vi "Final GUI for Team RDA.vi"() -> ()   [LabVIEW 2022 SP3]
doc: "This example is used to make the attitude control"
uses:
  GUI Animation/Fan.ctl
  GUI Animation/Dial.ctl
  GUI Animation/WiFi.ctl
  <vilib>/Platform/TimedLoop/XDataNode/timing_clust.ctl
  <vilib>/Platform/TimedLoop/XDataNode/nitl_modes.ctl
  <vilib>/Platform/TimedLoop/XDataNode/wakeup.ctl
  <vilib>/platform/TimedLoop/XDataNode/XDataNode.xnode
  Attitude Indicator/lv-attitudecontrol.lvlib
  <vilib>/Platform/TimedLoop/XDataNode/XDNodeRunTimeDep.lvlib
panel:
  in  "Command Roll 2":dbl
  in  "Command Pitch 2":dbl
  out "Command Yaw2":dbl
  in  "MotorROn":bool
  in  "MotorLON":bool
  out "?":bool
  out "JoyButton":bool
  out "MotorRightThrottle":dbl
  out "MotorLeftThrottle":dbl
  in  "Command Roll":dbl
  in  "Command Pitch":dbl
  in  "Command Yaw":dbl
  in  "RightPWM":dbl
  in  "LeftPWM":dbl
  in  "Control2ESP":bool
  in  "State Machine":i8
  out "Dialog":string
  in  "PC2ESP":bool
  out "WiFi 2":T1
  out "WiFi":T1
  out "Throttle":T2 scale=0.0..100.0
  out "Right Propeller":T3
  out "Left Propeller":T3
  out "Boolean 6":bool
  out "Yaw Displayed":i16
  out "Roll Displayed":dbl
  out "Boolean 3":bool
  in  "stop 4":bool
  out "Boolean 2":bool
  in  "stop 3":bool
  out "Pitch Displayed":dbl
  in  "Yaw":dbl min=0.0 max=360.0
  in  "Roll":dbl min=-180.0 max=180.0
  in  "Pitch":dbl min=-90.0 max=90.0
  in  "Attitude Indicator":refnum<vi>(3d-picture)
  in  "stop":bool
  # "pitch and roll from control"
types:
  T1 = typedef "WiFi.ctl" = u16
  T2 = typedef "Dial.ctl" = dbl
  T3 = typedef "Fan.ctl" = bool
  T4 = typedef "lv-attitudecontrol.lvlib/AttitudeHandle.ctl" = cluster{"First Scene Object":refnum<vi>, "Drum":refnum<vi>, "Window":refnum<vi>, "Dial":refnum<vi>, "Scene Graph":refnum<vi>, "Last Drum Pitch":dbl, "Last Drum Roll ":dbl, "Last Dial Roll":dbl}
  T5 = typedef "XDNodeRunTimeDep.lvlib/timing_clust.ctl" = cluster{"Expected End [f-1]":u64, "Actual End [f-1]":u64, "Finished Late? [f-1]":bool, "Expected End [i-1]":u64, "Actual End [i-1]":u64, "Finished Late? [i-1]":bool, "Expected Start [i]":u64, "Actual Start [i]":u64, "Expected Start [f]":u64, "Actual Start [f]":u64, "Source Name":string, "Structure Name":string, "Period":i64, "Deadline":i64, "Offset":i64, "Start":i64, "Priority":i32, "Timeout":i32, "Mode":T6, "Wakeup Reason":T7, "Error":errorcluster, "Source Type":string, "Secondary Source Type":string, "Global End Time":u64, "Global Start Time":u64, "Frame Duration":u64, "Iteration Duration":u64, "Assigned CPU":i32, "I/O Scan Engine Mode":u32}
  T6 = typedef "XDNodeRunTimeDep.lvlib/nitl_modes.ctl" = enum32{"No Change", "Process missed periods, maintain original phase", "Discard missed periods, maintain original phase", "Process missed periods, ignore original phase", "Discard missed periods, ignore original phase"}
  T7 = typedef "XDNodeRunTimeDep.lvlib/wakeup.ctl" = enum32{"Normal", "Aborted", "Asynchronous wakeup", "Timing source error", "Timed loop error", "Timeout"}
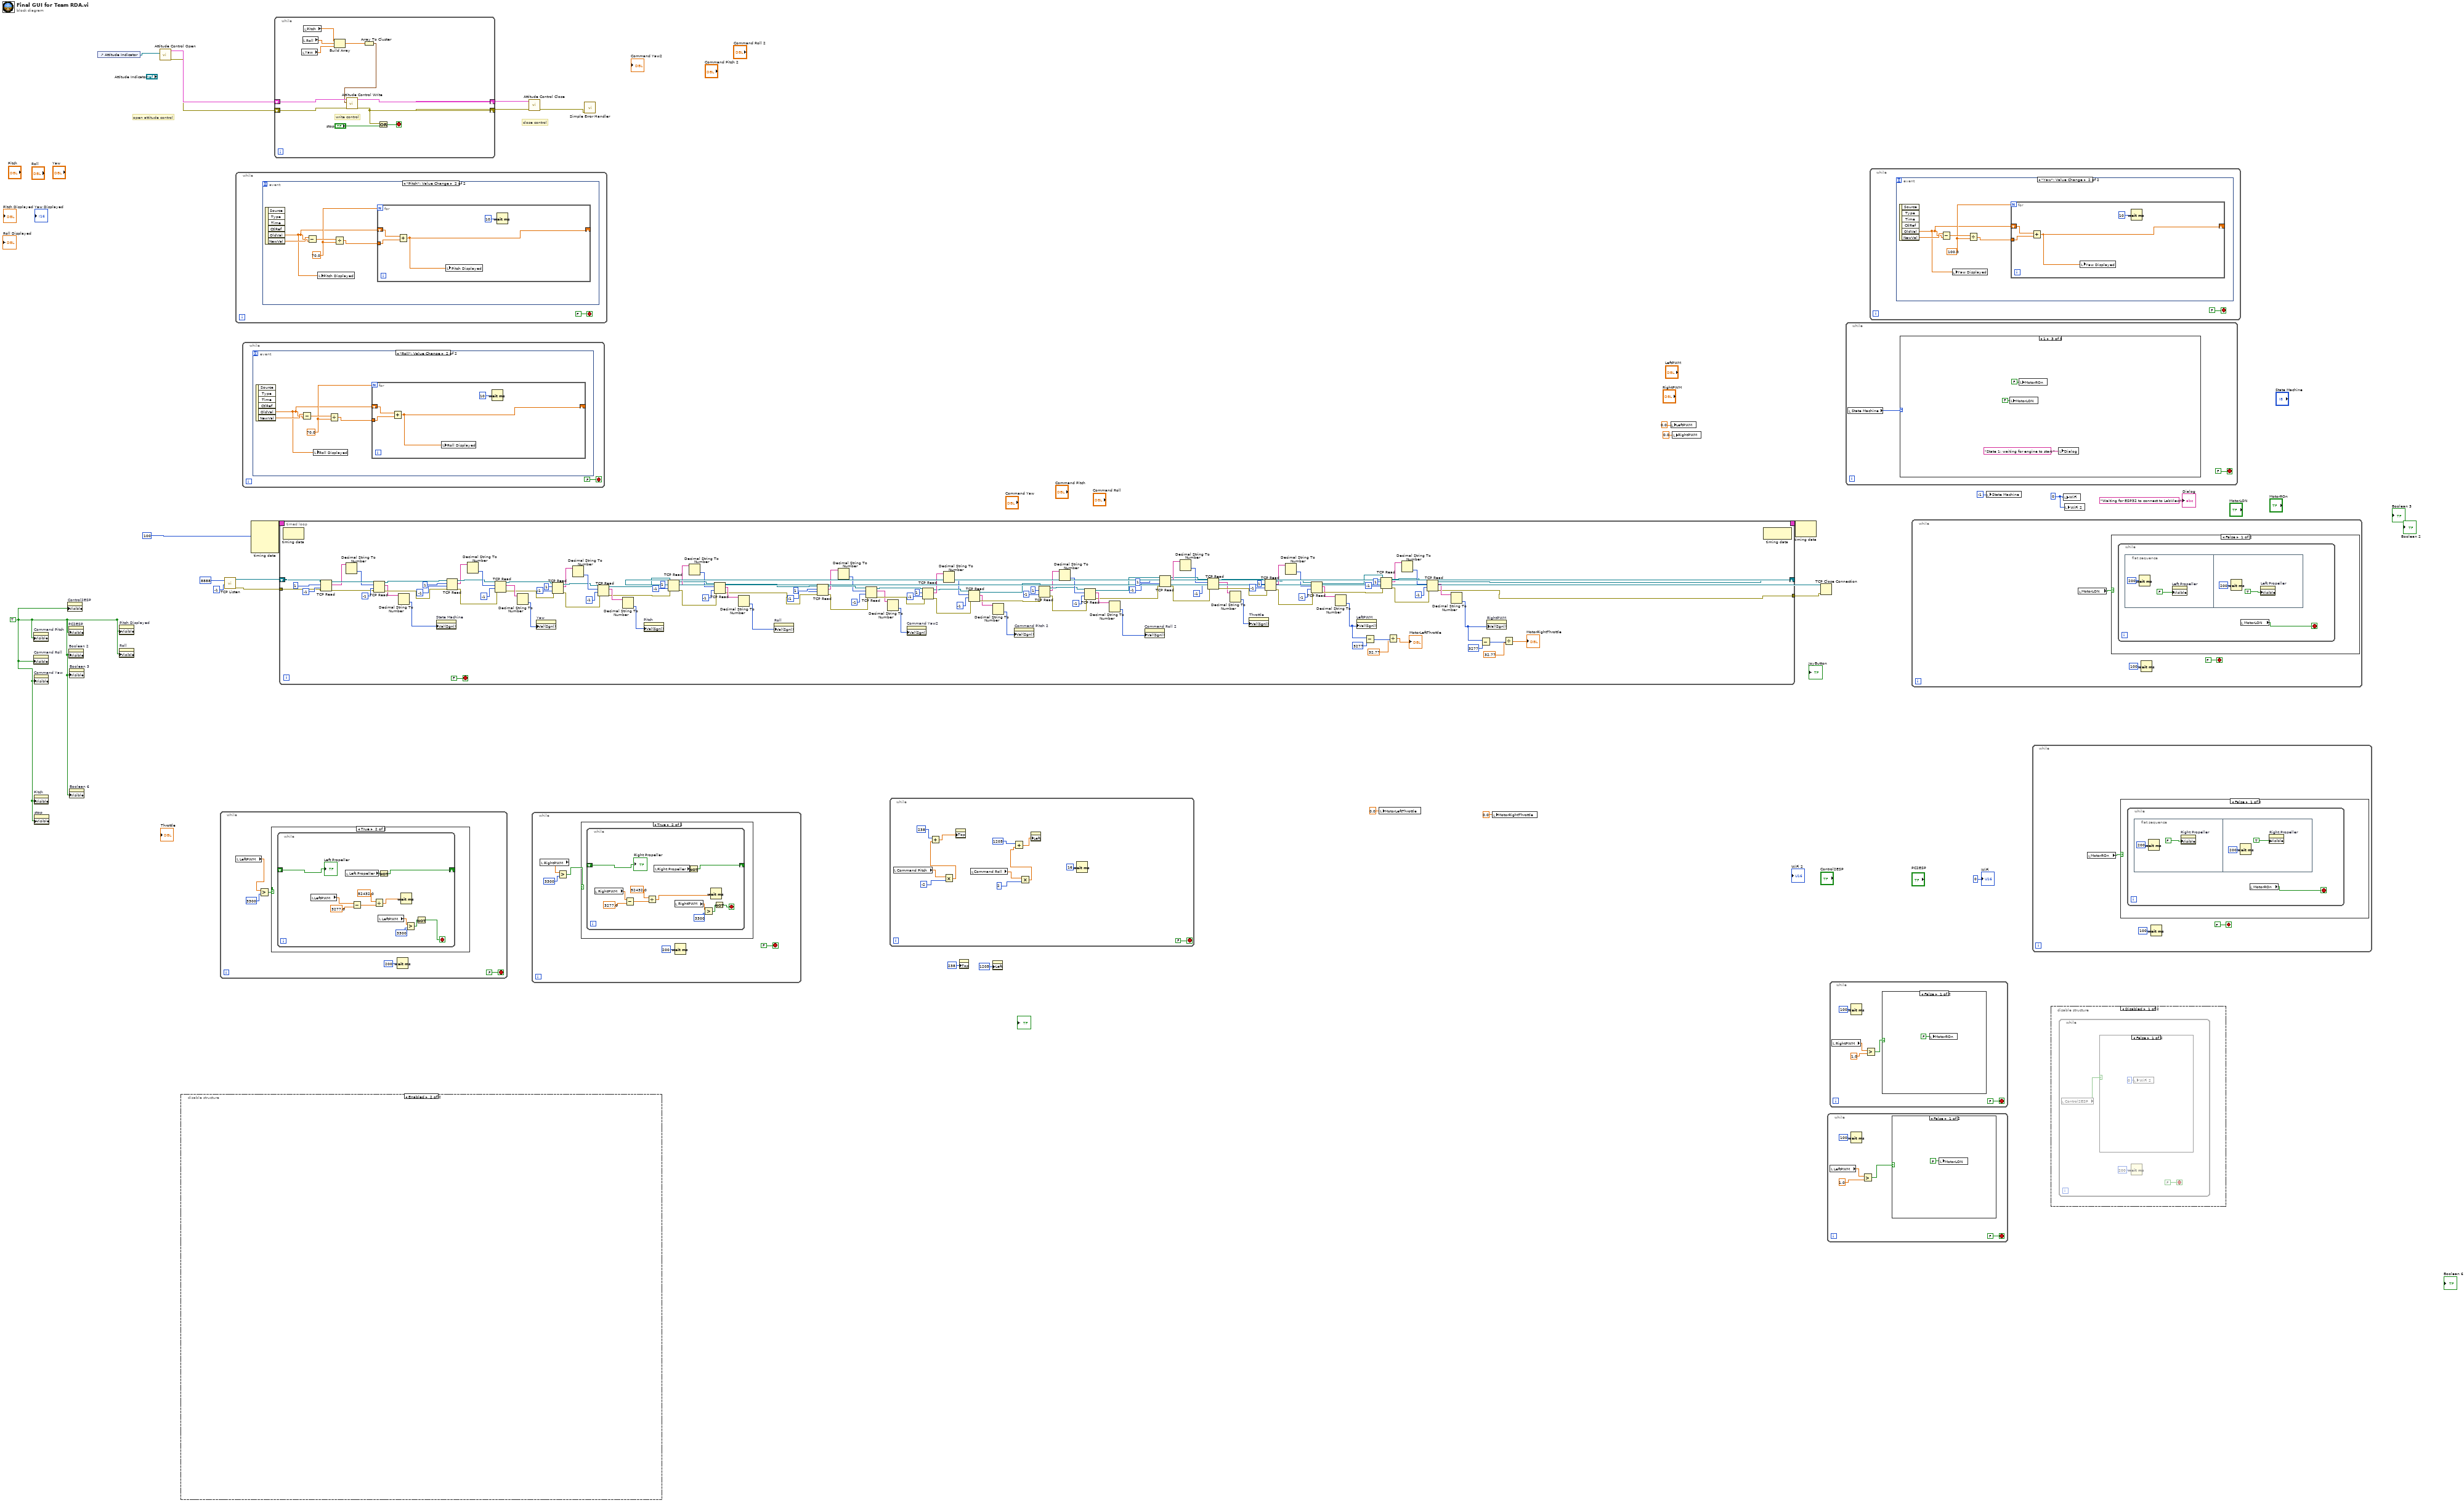
[diagram p0: block diagram]
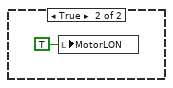
[diagram p2: hidden frame]
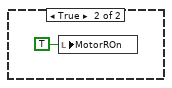
[diagram p3: hidden frame]
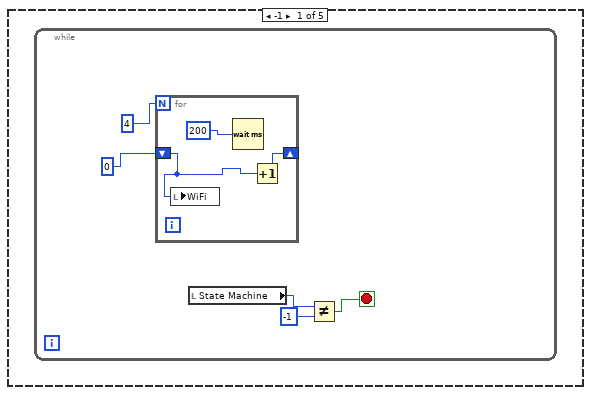
[diagram p8: hidden frame]
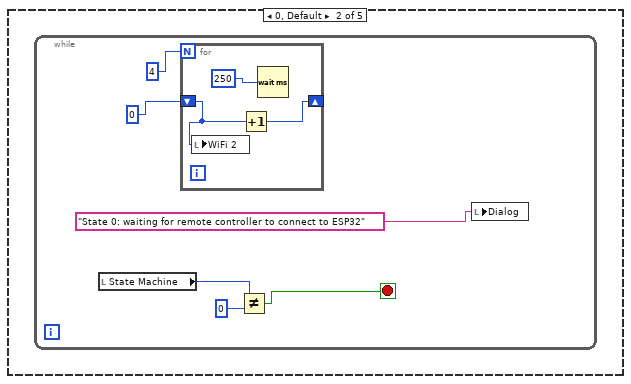
[diagram p9: hidden frame]
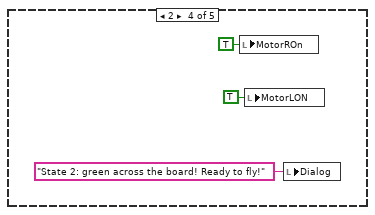
[diagram p10: hidden frame]
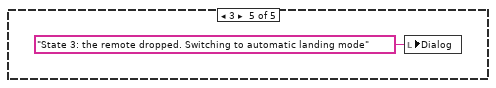
[diagram p11: hidden frame]
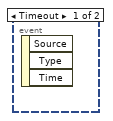
[diagram p14: hidden frame]
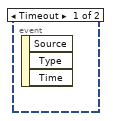
[diagram p15: hidden frame]
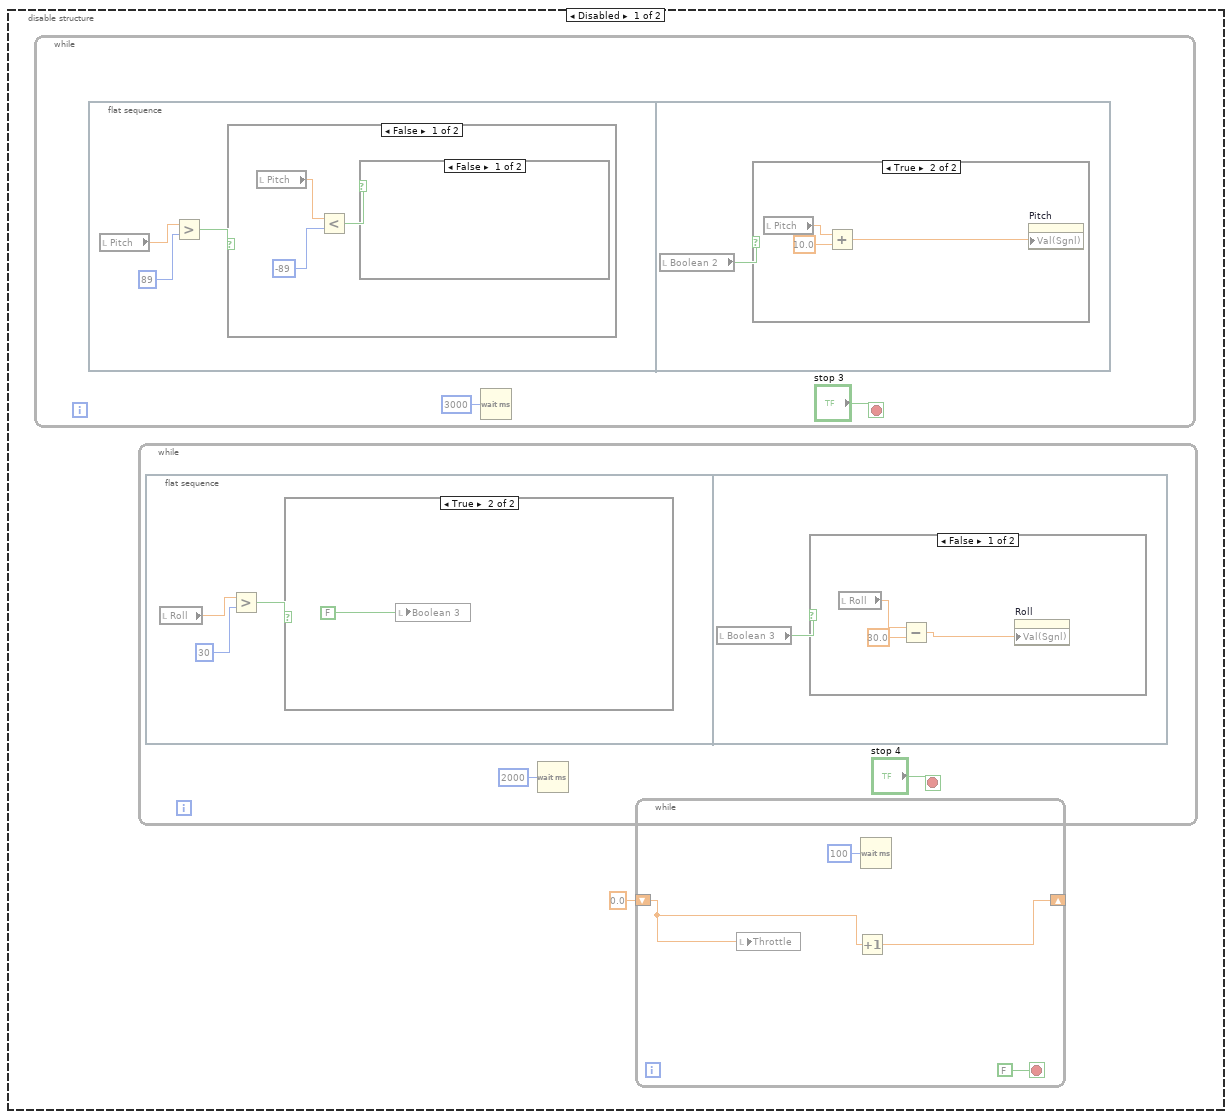
[diagram p16: hidden frame]
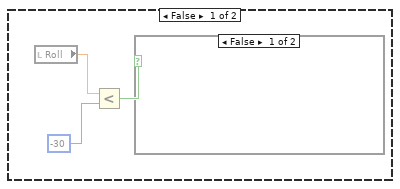
[diagram p17: hidden frame]
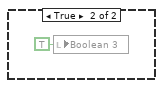
[diagram p18: hidden frame]
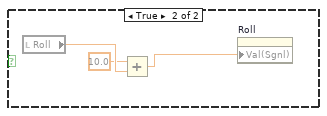
[diagram p19: hidden frame]
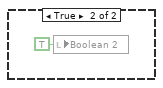
[diagram p20: hidden frame]
diagram:
  w5 = TRUE
  w10 = T1 0 ("WiFi")
  # "close control"
  # "open attitude control"
  n1 = property on="Command Pitch" class="DigNum (strict)"("Visible"=w5) -> ()  [unwired: 2 in, 2 out]
  n2 = property on="Command Roll" class="DigNum (strict)"("Visible"=w5) -> ()  [unwired: 2 in, 2 out]
  n3 = property on="Command Yaw" class="DigNum (strict)"("Visible"=w5) -> ()  [unwired: 2 in, 2 out]
  n4 = property on="Pitch" class="DigNum (strict)"("Visible"=w5) -> ()  [unwired: 2 in, 2 out]
  n5 = property on="stop" class="Bool"("Visible"=w5) -> ()  [unwired: 2 in, 2 out]
  n6 = property on="Control2ESP" class="Bool (strict)"("Visible"=w5) -> ()  [unwired: 2 in, 2 out]
  n7 = property on="PC2ESP" class="Bool (strict)"("Visible"=w5) -> ()  [unwired: 2 in, 2 out]
  n8 = property on="Boolean 2" class="Bool (strict)"("Visible"=w5) -> ()  [unwired: 2 in, 2 out]
  n9 = property on="Boolean 3" class="Bool (strict)"("Visible"=w5) -> ()  [unwired: 2 in, 2 out]
  n10 = property on="Boolean 6" class="Bool (strict)"("Visible"=w5) -> ()  [unwired: 2 in, 2 out]
  n11 = control-ref of="Attitude Indicator"() -> (w24:refnum<vi>)
  n12 = property on="Pitch Displayed" class="DigNum (strict)"("Visible"=w5) -> ()  [unwired: 2 in, 2 out]
  n13 = property on="Roll" class="DigNum (strict)"("Visible"=w5) -> ()  [unwired: 2 in, 2 out]
  n14 = call "Attitude Control Open.vi"("Scene Graph"=w24) -> ("error out"=w25:errorcluster, "Attitude Control Handle"=w26:T4)  [unwired: 9 in]
  n15 = disable-structure shown="Enabled" {
    frame Disabled {
      n16 = while {
        stop <- "stop 3" stop-if-true
        n17 = flat-sequence {
          frame #0 {
            n18 = local read "Pitch"() -> (w53:dbl)
            n19 = Greater?(x=w53, y=89) -> (0:w51:bool)
            n20 = case shown="False" w51 {
              frame False {
                n21 = local read "Pitch"() -> (w56:dbl)
                n22 = Less?(x=w56, y=-89) -> (x < y?=w54:bool)
                n23 = case shown="False" w54 {
                  frame False {
                  }
                  frame True {
                    n24 = local write "Boolean 2"(TRUE ("Boolean")) -> ()
                  }
                }
              }
              frame True {
                n25 = local write "Boolean 2"(FALSE ("Boolean")) -> ()
              }
            }
          }
          frame #1 {
            n26 = local read "Boolean 2"() -> (w59:bool)
            n27 = case shown="True" w59 {
              frame False {
                n28 = local read "Pitch"() -> (w62:dbl)
                n29 = Subtract(x=w62, y=10.0) -> (x-y=w60:dbl)
                n30 = property on="Pitch" class="DigNum (strict)"("Val(Sgnl)"=w60) -> ()  [unwired: 2 in, 2 out]
              }
              frame True {
                n31 = local read "Pitch"() -> (w65:dbl)
                n32 = Add(x=w65, y=10.0) -> (x+y=w63:dbl)
                n33 = property on="Pitch" class="DigNum (strict)"("Val(Sgnl)"=w63) -> ()  [unwired: 2 in, 2 out]
              }
            }
          }
        }
        n34 = Wait (ms)(milliseconds to wait=u32 3000) -> ()  [unwired: 1 out]
      }
      n35 = while {
        stop <- "stop 4" stop-if-true
        n36 = flat-sequence {
          frame #0 {
            n37 = local read "Roll"() -> (w36:dbl)
            n38 = Greater?(x=w36, y=30) -> (0:w34:bool)
            n39 = case shown="True" w34 {
              frame False {
                n40 = local read "Roll"() -> (w39:dbl)
                n41 = Less?(x=w39, y=-30) -> (x < y?=w37:bool)
                n42 = case shown="False" w37 {
                  frame False {
                  }
                  frame True {
                    n43 = local write "Boolean 3"(TRUE ("Boolean")) -> ()
                  }
                }
              }
              frame True {
                n44 = local write "Boolean 3"(FALSE ("Boolean")) -> ()
              }
            }
          }
          frame #1 {
            n45 = local read "Boolean 3"() -> (w42:bool)
            n46 = case shown="False" w42 {
              frame False {
                n47 = local read "Roll"() -> (w45:dbl)
                n48 = Subtract(x=w45, y=30.0) -> (x-y=w43:dbl)
                n49 = property on="Roll" class="DigNum (strict)"("Val(Sgnl)"=w43) -> ()  [unwired: 2 in, 2 out]
              }
              frame True {
                n50 = local read "Roll"() -> (w48:dbl)
                n51 = Add(x=10.0, y=w48) -> (x+y=w46:dbl)
                n52 = property on="Roll" class="DigNum (strict)"("Val(Sgnl)"=w46) -> ()  [unwired: 2 in, 2 out]
              }
            }
          }
        }
        n53 = Wait (ms)(milliseconds to wait=u32 2000) -> ()  [unwired: 1 out]
      }
      n54 = while {
        shift-right: [w29] -> _
        shift-left: 0.0 -> [w28]
        stop <- FALSE stop-if-true
        n55 = local write "Throttle"(w28) -> ()
        n56 = Increment(x=w28) -> (x+1=w29:dbl)
        n57 = Wait (ms)(milliseconds to wait=u32 100) -> ()  [unwired: 1 out]
      }
    }
    frame Enabled {
    }
  }
  n58 = while {
    stop <- FALSE stop-if-true
    n59 = local read "LeftPWM"() -> (w70:dbl)
    n60 = Greater?(x=w70, y=3300) -> (0:w69:bool)
    n61 = case shown="True" w69 {
      frame False {
      }
      frame True {
        n62 = while {
          shift-right: [w81] -> _
          shift-left: _ -> [w79]
          stop <- w80 stop-if-true
          n63 = local read "LeftPWM"() -> (w71:dbl)
          n64 = local read "Left Propeller"() -> (w82:T3)
          n65 = Subtract(x=w71, y=3277.0 ("x")) -> (x-y=w75:dbl)
          n66 = Divide(x=52432.0, y=w75) -> (x/y=w72:dbl)
          n67 = local read "LeftPWM"() -> (w76:dbl)
          n68 = Not(x=w82) -> (.not. x?=w81:T3)
          n69 = Wait (ms)(milliseconds to wait=w72) -> ()  [unwired: 1 out]
          n70 = Greater?(x=w76, y=3300) -> (0:w77:bool)
          n71 = Not(x=w77) -> (.not. x?=w80:bool)
          "Left Propeller" <- w79
        }
      }
    }
    n72 = Wait (ms)(milliseconds to wait=u32 200) -> ()  [unwired: 1 out]
  }
  n73 = call <vilib>:"TCP Listen.vi"("timeout ms (wait forever: -1)"=-1, "port"=u16 8888) -> ("error out"=w15:errorcluster, "connection ID"=w18:refnum<k5>)  [unwired: 5 in, 3 out]
  n74 = while {
    stop <- FALSE stop-if-true
    n75 = event shown="[1] \"Pitch\": Value Change" {
      selector: _ -> [_ _]
      dyn-events: _ -> [_ _]
      timeout: _ -> [_ _]
      event Timeout {
        n76 = event-data() -> ()  [unwired: 1 in, 3 out]
      }
      event "Pitch": Value Change {
        w86 = 70.0
        n77 = event-data() -> ("OldVal"=w84:dbl, "NewVal"=w88:dbl)  [unwired: 1 in, 4 out]
        n78 = Subtract(x=w88, y=w84) -> (x-y=w87:dbl)
        n79 = local write "Pitch Displayed"(w84) -> ()
        n80 = Divide(x=w87, y=w86) -> (x/y=w85:dbl)
        n81 = for {
          N: w86 -> [_]
          shift-right: [w89] -> _
          shift-left: w84 -> [w91]
          tunnel: w85 -> [w90]
          n82 = Add(x=w91, y=w90) -> (x+y=w89:dbl)
          n83 = local write "Pitch Displayed"(w89) -> ()
          n84 = Wait (ms)(milliseconds to wait=u32 10) -> ()  [unwired: 1 out]
        }
      }
    }
  }
  n85 = while {
    stop <- FALSE stop-if-true
    n86 = event shown="[1] \"Roll\": Value Change" {
      selector: _ -> [_ _]
      dyn-events: _ -> [_ _]
      timeout: _ -> [_ _]
      event Timeout {
        n87 = event-data() -> ()  [unwired: 1 in, 3 out]
      }
      event "Roll": Value Change {
        w96 = 70.0
        n88 = event-data() -> ("OldVal"=w94:dbl, "NewVal"=w98:dbl)  [unwired: 1 in, 4 out]
        n89 = Subtract(x=w98, y=w94) -> (x-y=w97:dbl)
        n90 = local write "Roll Displayed"(w94) -> ()
        n91 = Divide(x=w97, y=w96) -> (x/y=w95:dbl)
        n92 = for {
          N: w96 -> [_]
          shift-right: [w99] -> _
          shift-left: w94 -> [w101]
          tunnel: w95 -> [w100]
          n93 = Add(x=w101, y=w100) -> (x+y=w99:dbl)
          n94 = local write "Roll Displayed"(w99) -> ()
          n95 = Wait (ms)(milliseconds to wait=u32 10) -> ()  [unwired: 1 out]
        }
      }
    }
  }
  n96 = node-c288(i64 100 ("Period")) -> (w20:T5)  [unwired: 3 in]
  n97 = while {
    shift-right: [w108] -> w22
    shift-left: w26 -> [w113]
    shift-right: [w109] -> w23
    shift-left: w25 -> [w112]
    stop <- w110 stop-if-true
    # "write control"
    n98 = local read "Yaw"() -> (w106:dbl)
    n99 = local read "Roll"() -> (w107:dbl)
    n100 = local read "Pitch"() -> (w103:dbl)
    n101 = Build Array(w103, w107, w106) -> (w105:dbl[])
    n102 = Array To Cluster(array=w105) -> (cluster=w104:cluster{"[0]":dbl, "[1]":dbl, "[2]":dbl})
    n103 = call "Attitude Control Write.vi"("error in (no error)"=w112, "pitch (x), roll (y), yaw (z)"=w104, "Attitude Control Handle In"=w113) -> ("error out"=w109:errorcluster, "Attitude Control Handle Out"=w108:T4)  [unwired: 7 in]
    n104 = Or(x=w109, y="stop") -> (x .or. y?=w110:bool)
  }
  n105 = timed-loop {
    timing: w20 -> [_]
    timing-out: [_] -> w19
    shift-right: [w114] -> w14
    shift-left: w18 -> [w234]
    tunnel: w15 -> [w227]
    tunnel: [w115] -> w8
    stop <- FALSE stop-if-true
    n106 = node-c288() -> ()  [unwired: 1 in, 1 out]
    n107 = TCP Read(connection ID=w234, bytes to read=1, error in (no error)=w227, 9:-1 ("timeout ms (25000)")) -> (connection ID out=w231:refnum<k5>, data out=w230:string, error out=w226:errorcluster)  [unwired: 1 in]
    n108 = Decimal String To Number(string=w230) -> (number=w229:i32)  [unwired: 2 in, 1 out]
    n109 = TCP Read(connection ID=w231, bytes to read=w229, error in (no error)=w226, 9:-1 ("timeout ms (25000)")) -> (connection ID out=w222:refnum<k5>, data out=w216:string, error out=w221:errorcluster)  [unwired: 1 in]
    n110 = Decimal String To Number(string=w216) -> (number=w204:i32)  [unwired: 2 in, 1 out]
    n111 = property on="State Machine" class="DigNum (strict)"("Val(Sgnl)"=w204) -> ()  [unwired: 2 in, 2 out]
    n112 = TCP Read(connection ID=w222, bytes to read=1, error in (no error)=w221, 9:-1 ("timeout ms (25000)")) -> (connection ID out=w219:refnum<k5>, data out=w217:string, error out=w218:errorcluster)  [unwired: 1 in]
    n113 = Decimal String To Number(string=w217) -> (number=w224:i32)  [unwired: 2 in, 1 out]
    n114 = TCP Read(connection ID=w219, bytes to read=w224, error in (no error)=w218, 9:-1 ("timeout ms (25000)")) -> (connection ID out=w207:refnum<k5>, data out=w215:string, error out=w206:errorcluster)  [unwired: 1 in]
    n115 = Decimal String To Number(string=w215) -> (number=w203:i32)  [unwired: 2 in, 1 out]
    n116 = property on="Yaw" class="DigNum (strict)"("Val(Sgnl)"=w203) -> ()  [unwired: 2 in, 2 out]
    n117 = TCP Read(connection ID=w207, bytes to read=1, error in (no error)=w206, 9:-1 ("timeout ms (25000)")) -> (connection ID out=w212:refnum<k5>, data out=w210:string, error out=w211:errorcluster)  [unwired: 1 in]
    n118 = Decimal String To Number(string=w210) -> (number=w213:i32)  [unwired: 2 in, 1 out]
    n119 = TCP Read(connection ID=w212, bytes to read=w213, error in (no error)=w211, 9:-1 ("timeout ms (25000)")) -> (connection ID out=w193:refnum<k5>, data out=w205:string, error out=w192:errorcluster)  [unwired: 1 in]
    n120 = Decimal String To Number(string=w205) -> (number=w202:i32)  [unwired: 2 in, 1 out]
    n121 = property on="Pitch" class="DigNum (strict)"("Val(Sgnl)"=w202) -> ()  [unwired: 2 in, 2 out]
    n122 = TCP Read(connection ID=w193, bytes to read=1, error in (no error)=w192, 9:-1 ("timeout ms (25000)")) -> (connection ID out=w196:refnum<k5>, data out=w198:string, error out=w197:errorcluster)  [unwired: 1 in]
    n123 = Decimal String To Number(string=w198) -> (number=w195:i32)  [unwired: 2 in, 1 out]
    n124 = TCP Read(connection ID=w196, bytes to read=w195, error in (no error)=w197, 9:-1 ("timeout ms (25000)")) -> (connection ID out=w159:refnum<k5>, data out=w201:string, error out=w158:errorcluster)  [unwired: 1 in]
    n125 = Decimal String To Number(string=w201) -> (number=w191:i32)  [unwired: 2 in, 1 out]
    n126 = property on="Roll" class="DigNum (strict)"("Val(Sgnl)"=w191) -> ()  [unwired: 2 in, 2 out]
    n127 = TCP Read(connection ID=w159, bytes to read=1, error in (no error)=w158, 9:-1 ("timeout ms (25000)")) -> (connection ID out=w164:refnum<k5>, data out=w166:string, error out=w165:errorcluster)  [unwired: 1 in]
    n128 = Decimal String To Number(string=w166) -> (number=w161:i32)  [unwired: 2 in, 1 out]
    n129 = TCP Read(connection ID=w164, bytes to read=w161, error in (no error)=w165, 9:-1 ("timeout ms (25000)")) -> (connection ID out=w175:refnum<k5>, data out=w167:string, error out=w176:errorcluster)  [unwired: 1 in]
    n130 = Decimal String To Number(string=w167) -> (number=w178:i32)  [unwired: 2 in, 1 out]
    n131 = property on="Command Yaw2" class="DigNum (strict)"("Val(Sgnl)"=w178) -> ()  [unwired: 2 in, 2 out]
    n132 = TCP Read(connection ID=w175, bytes to read=1, error in (no error)=w176, 9:-1 ("timeout ms (25000)")) -> (connection ID out=w170:refnum<k5>, data out=w172:string, error out=w171:errorcluster)  [unwired: 1 in]
    n133 = Decimal String To Number(string=w172) -> (number=w169:i32)  [unwired: 2 in, 1 out]
    n134 = TCP Read(connection ID=w170, bytes to read=w169, error in (no error)=w171, 9:-1 ("timeout ms (25000)")) -> (connection ID out=w188:refnum<k5>, data out=w177:string, error out=w189:errorcluster)  [unwired: 1 in]
    n135 = Decimal String To Number(string=w177) -> (number=w179:i32)  [unwired: 2 in, 1 out]
    n136 = property on="Command Pitch 2" class="DigNum (strict)"("Val(Sgnl)"=w179) -> ()  [unwired: 2 in, 2 out]
    n137 = TCP Read(connection ID=w188, bytes to read=1, error in (no error)=w189, 9:-1 ("timeout ms (25000)")) -> (connection ID out=w185:refnum<k5>, data out=w183:string, error out=w184:errorcluster)  [unwired: 1 in]
    n138 = Decimal String To Number(string=w183) -> (number=w186:i32)  [unwired: 2 in, 1 out]
    n139 = TCP Read(connection ID=w185, bytes to read=w186, error in (no error)=w184, 9:-1 ("timeout ms (25000)")) -> (connection ID out=w128:refnum<k5>, data out=w180:string, error out=w127:errorcluster)  [unwired: 1 in]
    n140 = Decimal String To Number(string=w180) -> (number=w190:i32)  [unwired: 2 in, 1 out]
    n141 = property on="Command Roll 2" class="DigNum (strict)"("Val(Sgnl)"=w190) -> ()  [unwired: 2 in, 2 out]
    n142 = TCP Read(connection ID=w128, bytes to read=1, error in (no error)=w127, 9:-1 ("timeout ms (25000)")) -> (connection ID out=w133:refnum<k5>, data out=w135:string, error out=w134:errorcluster)  [unwired: 1 in]
    n143 = Decimal String To Number(string=w135) -> (number=w130:i32)  [unwired: 2 in, 1 out]
    n144 = TCP Read(connection ID=w133, bytes to read=w130, error in (no error)=w134, 9:-1 ("timeout ms (25000)")) -> (connection ID out=w144:refnum<k5>, data out=w136:string, error out=w145:errorcluster)  [unwired: 1 in]
    n145 = Decimal String To Number(string=w136) -> (number=w147:i32)  [unwired: 2 in, 1 out]
    n146 = property on="Throttle" class="Knob (strict)"("Val(Sgnl)"=w147) -> ()  [unwired: 2 in, 2 out]
    n147 = TCP Read(connection ID=w144, bytes to read=1, error in (no error)=w145, 9:-1 ("timeout ms (25000)")) -> (connection ID out=w139:refnum<k5>, data out=w141:string, error out=w140:errorcluster)  [unwired: 1 in]
    n148 = Decimal String To Number(string=w141) -> (number=w138:i32)  [unwired: 2 in, 1 out]
    n149 = TCP Read(connection ID=w139, bytes to read=w138, error in (no error)=w140, 9:-1 ("timeout ms (25000)")) -> (connection ID out=w156:refnum<k5>, data out=w146:string, error out=w157:errorcluster)  [unwired: 1 in]
    n150 = Decimal String To Number(string=w146) -> (number=w126:i32)  [unwired: 2 in, 1 out]
    n151 = property on="LeftPWM" class="DigNum (strict)"("Val(Sgnl)"=w126) -> ()  [unwired: 2 in, 2 out]
    n152 = Subtract(x=w126, y=3277) -> (x-y=w124:i32)
    n153 = TCP Read(connection ID=w156, bytes to read=1, error in (no error)=w157, 9:-1 ("timeout ms (25000)")) -> (connection ID out=w153:refnum<k5>, data out=w151:string, error out=w152:errorcluster)  [unwired: 1 in]
    n154 = Divide(x=w124, y=32.77) -> (x/y=→"MotorLeftThrottle":dbl)
    n155 = Decimal String To Number(string=w151) -> (number=w154:i32)  [unwired: 2 in, 1 out]
    n156 = TCP Read(connection ID=w153, bytes to read=w154, error in (no error)=w152, 9:-1 ("timeout ms (25000)")) -> (connection ID out=w114:refnum<k5>, data out=w148:string, error out=w115:errorcluster)  [unwired: 1 in]
    n157 = Decimal String To Number(string=w148) -> (number=w118:i32)  [unwired: 2 in, 1 out]
    n158 = Subtract(x=w118, y=3277) -> (x-y=w120:i32)
    n159 = property on="RightPWM" class="DigNum (strict)"("Val(Sgnl)"=w118) -> ()  [unwired: 2 in, 2 out]
    n160 = Divide(x=w120, y=32.77) -> (x/y=→"MotorRightThrottle":dbl)
    n161 = node-c288() -> ()  [unwired: 1 in, 1 out]
  }
  n162 = call "Attitude Control Close.vi"("error in (no error)"=w23, "Attitude Control Handle"=w22) -> ("error out"=w21:errorcluster)  [unwired: 9 in]
  n163 = while {
    stop <- FALSE stop-if-true
    n164 = local read "RightPWM"() -> (w241:dbl)
    n165 = Greater?(x=w241, y=3300) -> (0:w240:bool)
    n166 = case shown="True" w240 {
      frame False {
      }
      frame True {
        n167 = while {
          shift-right: [w252] -> _
          shift-left: _ -> [w250]
          stop <- w251 stop-if-true
          n168 = local read "RightPWM"() -> (w245:dbl)
          n169 = Subtract(x=w245, y=3277.0 ("x")) -> (x-y=w242:dbl)
          n170 = Divide(x=52432.0, y=w242) -> (x/y=w246:dbl)
          n171 = local read "Right Propeller"() -> (w253:T3)
          n172 = local read "RightPWM"() -> (w247:dbl)
          n173 = Not(x=w253) -> (.not. x?=w252:T3)
          n174 = Greater?(x=w247, y=3300) -> (0:w248:bool)
          n175 = Wait (ms)(milliseconds to wait=w246) -> ()  [unwired: 1 out]
          n176 = Not(x=w248) -> (.not. x?=w251:bool)
          "Right Propeller" <- w250
        }
      }
    }
    n177 = Wait (ms)(milliseconds to wait=u32 200) -> ()  [unwired: 1 out]
  }
  n178 = call <vilib>:"Simple Error Handler.vi"("error in (no error)"=w21) -> ()  [unwired: 4 in, 5 out]
  n179 = while {
    stop <- FALSE stop-if-true
    n180 = local read "Command Pitch"() -> (w261:dbl)
    n181 = Multiply(x=w261, y=-2) -> (x*y=w262:dbl)
    n182 = Add(x=238 ("Position:Left"), y=w262) -> (x+y=w257:dbl)
    n183 = property class="Bool (strict)"("Top"=w257) -> ()  [unwired: 2 in, 2 out]
    n184 = local read "Command Roll"() -> (w258:dbl)
    n185 = Multiply(x=w258, y=2) -> (x*y=w254:dbl)
    n186 = Add(x=1205 ("Position:Top"), y=w254) -> (x+y=w256:dbl)
    n187 = property class="Bool (strict)"("Left"=w256) -> ()  [unwired: 2 in, 2 out]
    n188 = Wait (ms)(milliseconds to wait=u32 16) -> ()  [unwired: 1 out]
  }
  n189 = property class="Bool (strict)"("Top"=238 ("Position:Top")) -> ()  [unwired: 2 in, 2 out]
  n190 = property class="Bool (strict)"("Left"=1205 ("Position:Left")) -> ()  [unwired: 2 in, 2 out]
  n191 = local write "MotorLeftThrottle"(0.0 ("MotorLeftThrottle")) -> ()
  n192 = local write "MotorRightThrottle"(0.0 ("MotorRightThrottle")) -> ()
  n193 = local write "LeftPWM"(0.0 ("LeftPWM")) -> ()
  n194 = local write "RightPWM"(0.0 ("RightPWM")) -> ()
  n195 = node-c288(w19) -> ()  [unwired: 1 out]
  n196 = TCP Close Connection(connection ID=w14, error in (no error)=w8) -> ()  [unwired: 1 in, 2 out]
  n197 = while {
    stop <- FALSE stop-if-true
    n198 = local read "LeftPWM"() -> (w269:dbl)
    n199 = Wait (ms)(milliseconds to wait=u32 100) -> ()  [unwired: 1 out]
    n200 = Greater?(x=w269, y=1.0) -> (0:w270:bool)
    n201 = case shown="False" w270 {
      frame False {
        n202 = local write "MotorLON"(FALSE ("MotorLON")) -> ()
      }
      frame True {
        n203 = local write "MotorLON"(TRUE ("MotorLON")) -> ()
      }
    }
  }
  n204 = while {
    stop <- FALSE stop-if-true
    n205 = local read "RightPWM"() -> (w277:dbl)
    n206 = Wait (ms)(milliseconds to wait=u32 100) -> ()  [unwired: 1 out]
    n207 = Greater?(x=w277, y=1.0) -> (0:w276:bool)
    n208 = case shown="False" w276 {
      frame False {
        n209 = local write "MotorROn"(FALSE ("MotorLON")) -> ()
      }
      frame True {
        n210 = local write "MotorROn"(TRUE ("MotorLON")) -> ()
      }
    }
  }
  n211 = while {
    stop <- FALSE stop-if-true
    n212 = local read "State Machine"() -> (w280:i8)
    n213 = case shown="1" w280 {
      frame -1 {
        n214 = while {
          stop <- w285 stop-if-true
          n215 = for {
            N: 4 -> [_]
            shift-right: [w288] -> _
            shift-left: 0 -> [w287]
            n216 = local write "WiFi"(w287) -> ()
            n217 = Wait (ms)(milliseconds to wait=u32 200 ("millisecond timer value")) -> ()  [unwired: 1 out]
            n218 = Increment(x=w287) -> (x+1=w288:i32)
          }
          n219 = local read "State Machine"() -> (w286:i8)
          n220 = Not Equal?(x=w286, y=i8 -1) -> (x != y?=w285:bool)
        }
      }
      frame 0, Default {
        n221 = while {
          stop <- w293 stop-if-true
          n222 = local read "State Machine"() -> (w292:i8)
          n223 = for {
            N: 4 -> [_]
            shift-right: [w296] -> _
            shift-left: 0 -> [w297]
            n224 = local write "WiFi 2"(w297) -> ()
            n225 = Increment(x=w297) -> (x+1=w296:i32)
            n226 = Wait (ms)(milliseconds to wait=u32 250 ("millisecond timer value")) -> ()  [unwired: 1 out]
          }
          n227 = Not Equal?(x=w292, y=i8 0) -> (x != y?=w293:bool)
          n228 = local write "Dialog"("State 0: waiting for remote controller to connect to ESP32" ("Dialog")) -> ()
        }
      }
      frame 1 {
        n229 = local write "MotorLON"(FALSE ("MotorON")) -> ()
        n230 = local write "MotorROn"(FALSE ("MotorON")) -> ()
        n231 = local write "Dialog"("State 1: waiting for engine to start " ("Dialog")) -> ()
      }
      frame 2 {
        n232 = local write "MotorROn"(TRUE ("MotorON")) -> ()
        n233 = local write "MotorLON"(TRUE ("MotorON")) -> ()
        n234 = local write "Dialog"("State 2: green across the board! Ready to fly!" ("Dialog")) -> ()
      }
      frame 3 {
        n235 = local write "Dialog"("State 3: the remote dropped. Switching to automatic landing mode" ("Dialog")) -> ()
      }
    }
  }
  n236 = while {
    stop <- FALSE stop-if-true
    n237 = event shown="[1] \"Yaw\": Value Change" {
      selector: _ -> [_ _]
      dyn-events: _ -> [_ _]
      timeout: _ -> [_ _]
      event Timeout {
        n238 = event-data() -> ()  [unwired: 1 in, 3 out]
      }
      event "Yaw": Value Change {
        w309 = 100.0
        n239 = event-data() -> ("OldVal"=w307:dbl, "NewVal"=w311:dbl)  [unwired: 1 in, 4 out]
        n240 = Subtract(x=w311, y=w307) -> (x-y=w310:dbl)
        n241 = local write "Yaw Displayed"(w307) -> ()
        n242 = Divide(x=w310, y=w309) -> (x/y=w308:dbl)
        n243 = for {
          N: w309 -> [_]
          shift-right: [w312] -> _
          shift-left: w307 -> [w314]
          tunnel: w308 -> [w313]
          n244 = Add(x=w314, y=w313) -> (x+y=w312:dbl)
          n245 = local write "Yaw Displayed"(w312) -> ()
          n246 = Wait (ms)(milliseconds to wait=u32 10) -> ()  [unwired: 1 out]
        }
      }
    }
  }
  n247 = while {
    stop <- FALSE stop-if-true
    n248 = local read "MotorLON"() -> (w316:bool)
    n249 = case shown="False" w316 {
      frame False {
        n250 = while {
          stop <- w319 stop-if-true
          n251 = flat-sequence {
            frame #0 {
              n252 = Wait (ms)(milliseconds to wait=u32 200) -> ()  [unwired: 1 out]
              n253 = property on="Left Propeller" class="Bool (strict)"("Visible"=FALSE) -> ()  [unwired: 2 in, 2 out]
            }
            frame #1 {
              n254 = Wait (ms)(milliseconds to wait=u32 200) -> ()  [unwired: 1 out]
              n255 = property on="Left Propeller" class="Bool (strict)"("Visible"=TRUE) -> ()  [unwired: 2 in, 2 out]
            }
          }
          n256 = local read "MotorLON"() -> (w319:bool)
        }
      }
      frame True {
      }
    }
    n257 = Wait (ms)(milliseconds to wait=u32 100) -> ()  [unwired: 1 out]
  }
  n258 = local write "State Machine"(i8 -1 ("State Machine")) -> ()
  n259 = while {
    stop <- FALSE stop-if-true
    n260 = local read "MotorROn"() -> (w324:bool)
    n261 = case shown="False" w324 {
      frame False {
        n262 = while {
          stop <- w327 stop-if-true
          n263 = flat-sequence {
            frame #0 {
              n264 = Wait (ms)(milliseconds to wait=u32 200) -> ()  [unwired: 1 out]
              n265 = property on="Right Propeller" class="Bool (strict)"("Visible"=FALSE) -> ()  [unwired: 2 in, 2 out]
            }
            frame #1 {
              n266 = Wait (ms)(milliseconds to wait=u32 200) -> ()  [unwired: 1 out]
              n267 = property on="Right Propeller" class="Bool (strict)"("Visible"=TRUE) -> ()  [unwired: 2 in, 2 out]
            }
          }
          n268 = local read "MotorROn"() -> (w327:bool)
        }
      }
      frame True {
      }
    }
    n269 = Wait (ms)(milliseconds to wait=u32 100) -> ()  [unwired: 1 out]
  }
  n270 = disable-structure shown="Disabled" {
    frame Disabled {
      n271 = while {
        stop <- FALSE stop-if-true
        n272 = local read "Control2ESP"() -> (w333:bool)
        n273 = case shown="False" w333 {
          frame False {
            n274 = local write "WiFi 2"(T1 0 ("WiFi")) -> ()
          }
          frame True {
          }
        }
        n275 = Wait (ms)(milliseconds to wait=u32 200) -> ()  [unwired: 1 out]
      }
    }
    frame Enabled {
    }
  }
  n276 = local write "WiFi"(w10) -> ()
  n277 = local write "WiFi 2"(w10) -> ()
  "WiFi" <- T1 0 ("WiFi")
  "Dialog" <- "Waiting for ESP32 to connect to LabView" ("Dialog")
